vi "fgv_PwrPak7-232.vi"(7 "cmd":T1, 8 "error in":errorcluster, 10 "baud rate":u32=115200) -> (0 "error out":errorcluster, 1 "null time":dbl, 2 "buff":u32, 3 "read data":string)   [LabVIEW 2019]
uses:
  Ctrl/gps-232.ctl
  <vilib>/Instr/_visa.llb/VISA Set IO Buffer Mask.ctl
  <vilib>/Instr/_visa.llb/VISA Configure Serial Port (Instr).vi
panel:
  in  "GNSSLogCMD":string
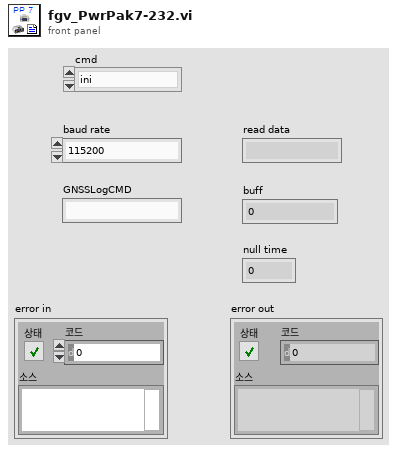
[diagram p1: front panel]
types:
  T1 = typedef "gps-232.ctl" = enum16{"ini", "timing set", "read", "write", "close"}
  T2 = typedef "VISA Set IO Buffer Mask.ctl" = u16
  T3 = typedef "gnss_config.ctl" = cluster{"Port":refnum<visa-resource-name>, "heading select":string, "PwrPak7_mode select":string[], "rate":u32}
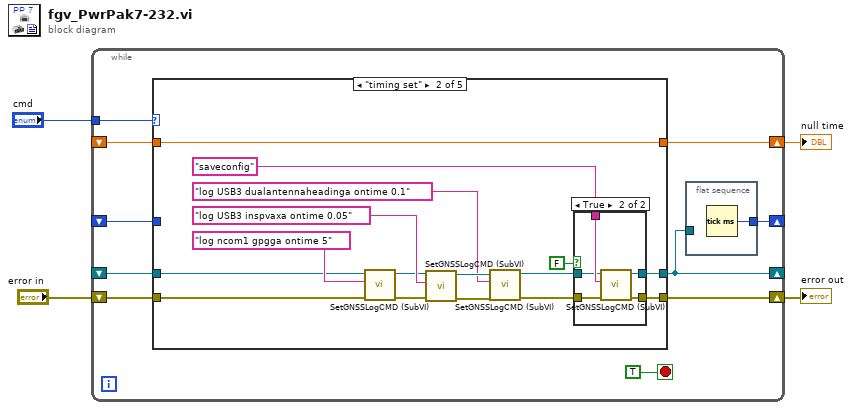
[diagram p0: block diagram]
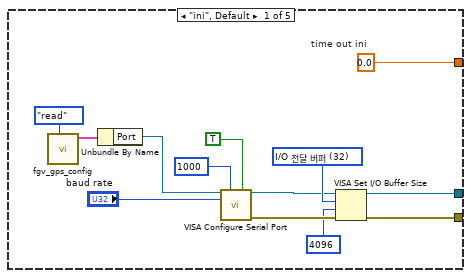
[diagram p2: hidden frame]
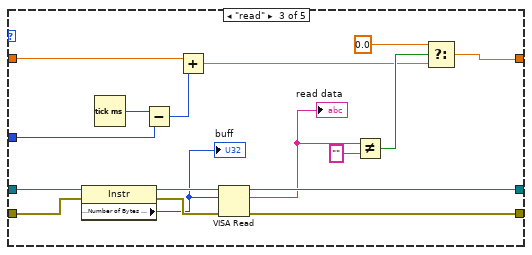
[diagram p4: hidden frame]
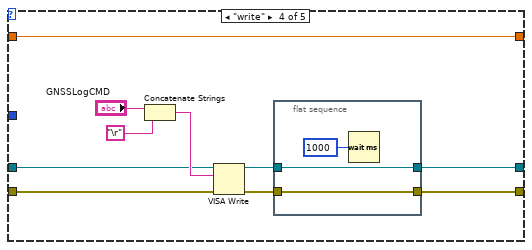
[diagram p5: hidden frame]
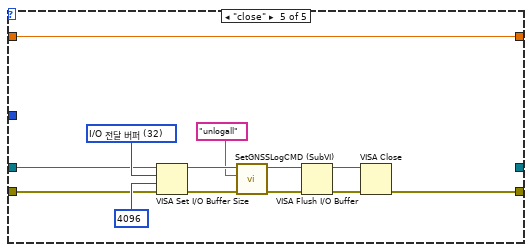
[diagram p6: hidden frame]
diagram:
  n1 = while {
    shift-right: [w13] -> w3
    shift-left: "error in" -> [w11]
    shift-right: [w5] -> _
    shift-left: _ -> [w10]
    tunnel: "cmd" -> [w12]
    shift-right: [w6] -> w1
    shift-left: _ -> [w9]
    shift-right: [w8] -> _
    shift-left: _ -> [w7]
    stop <- TRUE stop-if-true
    n2 = case shown="\"timing set\"" w12 {
      tunnel: [w21 w33 w64 w70 w83] -> w13
      tunnel: [w22 w32 w65 w71 _] -> w5
      tunnel: w11 -> [_ w37 w62 w73 w84]
      tunnel: w10 -> [_ w31 w63 w72 w85]
      tunnel: [w20 w30 w58 w69 w82] -> w6
      tunnel: w9 -> [_ w30 w54 w69 w82]
      tunnel: w7 -> [_ _ w55 _ _]
      frame "ini", Default {
        w20 = 0.0  # time out ini
        w26 = T2 32 items=["I/O 받기 버퍼"=16, "I/O 전달 버퍼"=32, "I/O 받기와 전달 버퍼"=48] ("Mask")
        n3 = call "fgv_gps_config.vi"("cmd"=enum16{"read", "write"}."read") -> ("GNSS cfg out"=w17:T3)  [unwired: 9 in, 1 out]
        n4 = Unbundle By Name(w17) -> ("Port"=w16:refnum<visa-resource-name>)
        n5 = call-poly "VISA Configure Serial Port"("VISA resource name"=w16, "timeout (10sec)"=u32 1000, "Enable Termination\nChar (T)"=TRUE ("enable termination char"), "baud rate (9600)"="baud rate") -> ("VISA resource name out"=w23:refnum<visa-resource-name>, "error out"=w28:errorcluster)  [unwired: 10 in]
        n6 = VISA Set I/O Buffer Size(VISA resource name=w23, mask (16)=w26, size (4096)=u32 4096 ("크기(4096)"), error in (no error)=w28) -> (VISA resource name out=w22:refnum<visa-resource-name>, error out=w21:errorcluster)
      }
      frame "timing set" {
        n7 = call "SetGNSSLogCMD (SubVI).vi"("VISA"=w31, "GNSSLogCMD"="log ncom1 gpgga ontime 5" ("write buffer"), "error in"=w37) -> ("VISA out"=w39:refnum<visa-resource-name>, "error out"=w36:errorcluster)  [unwired: 6 in]
        n8 = call "SetGNSSLogCMD (SubVI).vi"("VISA"=w39, "GNSSLogCMD"="log USB3 inspvaxa ontime 0.05" ("write buffer"), "error in"=w36) -> ("VISA out"=w43:refnum<visa-resource-name>, "error out"=w35:errorcluster)  [unwired: 6 in]
        n9 = call "SetGNSSLogCMD (SubVI).vi"("VISA"=w43, "GNSSLogCMD"="log USB3 dualantennaheadinga ontime 0.1" ("write buffer"), "error in"=w35) -> ("VISA out"=w41:refnum<visa-resource-name>, "error out"=w34:errorcluster)  [unwired: 6 in]
        n10 = case shown="True" FALSE {
          tunnel: "saveconfig" ("write buffer") -> [_ w51]
          tunnel: w41 -> [w46 w50]
          tunnel: w34 -> [w45 w49]
          tunnel: [w45 w48] -> w33
          tunnel: [w46 w47] -> w32
          frame False {
          }
          frame True {
            n11 = call "SetGNSSLogCMD (SubVI).vi"("VISA"=w50, "GNSSLogCMD"=w51, "error in"=w49) -> ("VISA out"=w47:refnum<visa-resource-name>, "error out"=w48:errorcluster)  [unwired: 6 in]
          }
        }
      }
      frame "read" {
        n12 = property class="Instr"(reference=w63, error in=w62) -> (reference out=w67:refnum<visa-resource-name>, error out=w68:errorcluster, "Serial Settings:Number of Bytes at Serial Port"=w66:u32)
        "buff" <- w66
        n13 = Tick Count (ms)() -> (millisecond timer value=w56:u32)
        n14 = Subtract(x=w56, y=w55) -> (x-y=w53:u32)
        n15 = Add(x=w54, y=w53) -> (x+y=w52:dbl)
        n16 = VISA Read(VISA resource name=w67, byte count=w66, error in (no error)=w68) -> (VISA resource name out=w65:refnum<visa-resource-name>, read buffer=w61:string, error out=w64:errorcluster)  [unwired: 1 out]
        "read data" <- w61
        n17 = Not Equal?(x=w61, y="") -> (x != y?=w59:bool)
        n18 = Select(t=0.0, s=w59, f=w52) -> (s? t:f=w58:dbl)
      }
      frame "write" {
        n19 = Concatenate Strings("GNSSLogCMD", "\r") -> (w76:string)
        n20 = VISA Write(VISA resource name=w72, write buffer=w76, error in (no error)=w73) -> (VISA resource name out=w75:refnum<visa-resource-name>, error out=w74:errorcluster)  [unwired: 1 out]
        n21 = flat-sequence {
          tunnel: [w80] -> w71
          tunnel: w75 -> [w80]
          tunnel: w74 -> [w79]
          tunnel: [w79] -> w70
          frame #0 {
            n22 = Wait (ms)(milliseconds to wait=u32 1000) -> ()  [unwired: 1 out]
          }
        }
      }
      frame "close" {
        w91 = T2 32 items=["I/O 받기 버퍼"=16, "I/O 전달 버퍼"=32, "I/O 받기와 전달 버퍼"=48] ("Mask")
        n23 = VISA Set I/O Buffer Size(VISA resource name=w85, mask (16)=w91, size (4096)=u32 4096 ("크기(4096)"), error in (no error)=w84) -> (VISA resource name out=w89:refnum<visa-resource-name>, error out=w90:errorcluster)
        n24 = call "SetGNSSLogCMD (SubVI).vi"("VISA"=w89, "GNSSLogCMD"="unlogall" ("write buffer"), "error in"=w90) -> ("VISA out"=w93:refnum<visa-resource-name>, "error out"=w94:errorcluster)  [unwired: 6 in]
        n25 = VISA Flush I/O Buffer(VISA resource name=w93, error in (no error)=w94) -> (VISA resource name out=w86:refnum<visa-resource-name>, error out=w87:errorcluster)  [unwired: 1 in]
        n26 = VISA Close(VISA resource name=w86, error in (no error)=w87) -> (error out=w83:errorcluster)
      }
    }
    n27 = flat-sequence {
      tunnel: [w15] -> w8
      tunnel: w5 -> [_]
      frame #0 {
        n28 = Tick Count (ms)() -> (millisecond timer value=w15:u32)
      }
    }
  }
  "error out" <- w3
  "null time" <- w1
